vi "tcpDeviceMainExample.vi"() -> ()   [LabVIEW 2016]
uses:
  typedefs/deviceStatus.ctl
  typedefs/statusEnum.ctl
  ts_labview_tcp/tcpTypedefs/TCPSettings.ctl
  ExampleDevice/tcpExampleControler.lvclass
panel:
  out "timeout?":bool
  out "status":T1
  in  "stop":bool
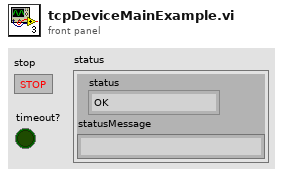
[diagram p1: front panel]
types:
  T1 = typedef "deviceStatus.ctl" = cluster{"status":T2, "statusMessage":string}
  T2 = typedef "statusEnum.ctl" = enum16{"OK", "TIMEOUT", "MSGERROR"}
  T3 = typedef "TCPSettings.ctl" = cluster{"IP":string, "port_low":u16, "port_up":u16, "connection_timeout ":i32, "reading_timeout":i32, "writing_timeout":i32}
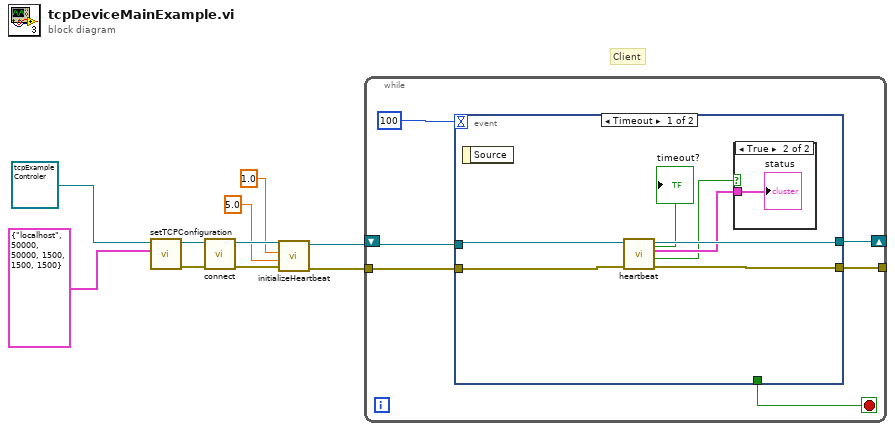
[diagram p0: block diagram]
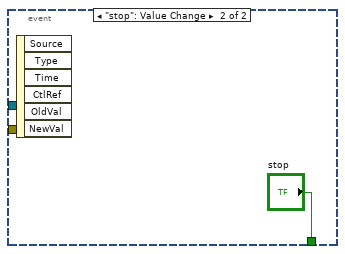
[diagram p3: hidden frame]
diagram:
  # "Client"
  n1 = call-dynamic "setTCPConfiguration.vi"("Settings"=T3 {"IP"="localhost", "port_low"=50000, "port_up"=50000, "connection_timeout "=1500, "reading_timeout"=1500, "writing_timeout"=1500}, "tcpDevice in"=refnum<class "tcpExampleControler.lvclass"> refnum ("tcpExampleControler.lvclass")) -> ("error out"=w8:errorcluster, "tcpDevice out"=w9:refnum<class "tcpExampleControler.lvclass">)  [unwired: 8 in]
  n2 = call-dynamic "connect.vi"("error in (no error)"=w8, "tcpDevice in"=w9) -> ("error out"=w6:errorcluster, "tcpDevice out"=w7:refnum<class "tcpExampleControler.lvclass">)  [unwired: 8 in]
  n3 = call-dynamic "initializeHeartbeat.vi"("error in (no error)"=w6, "timeout"=5.0, "period"=1.0, "tcpDevice in"=w7) -> ("error out"=w5:errorcluster, "tcpDevice out"=w4:refnum<class "tcpExampleControler.lvclass">)  [unwired: 6 in]
  n4 = while {
    tunnel: w5 -> [w13]
    shift-right: [w12] -> _
    shift-left: w4 -> [w14]
    tunnel: [w11] -> _
    stop <- w15 stop-if-true
    n5 = event shown="[0] Timeout" {
      selector: _ -> [_ _]
      dyn-events: _ -> [_ _]
      timeout: 100 -> [_ _]
      tunnel: [_ "stop"] -> w15
      tunnel: w14 -> [w23 _]
      tunnel: w13 -> [w19 _]
      tunnel: [w20 _] -> w11
      tunnel: [w22 _] -> w12
      event Timeout {
        n6 = event-data() -> ()  [unwired: 1 in, 1 out]
        n7 = call-dynamic "heartbeat.vi"("error in (no error)"=w19, "tcpDevice in"=w23) -> ("error out"=w20:errorcluster, "newValue"=w17:bool, "status"=w21:T1, "tcpDevice out"=w22:refnum<class "tcpExampleControler.lvclass">, "timeout?"=→"timeout?":bool)  [unwired: 5 in]
        n8 = case shown="True" w17 {
          tunnel: w21 -> [_ w24]
          frame False {
          }
          frame True {
            "status" <- w24
          }
        }
      }
      event "stop": Value Change {
        n9 = event-data() -> ()  [unwired: 1 in, 6 out]
      }
    }
  }
